vi "IsSearchGoalNode.vi"(8 "error in (no error)":errorcluster, 10 "NodeToIdentify in":refnum<data-value>, 11 "BasicSortedList in":refnum<class "BasicSortedList.lvclass">) -> (0 "error out":errorcluster, 1 "IsNode":bool, 2 "NodeToIdentify out":refnum<data-value>, 3 "BasicSortedList out":refnum<class "BasicSortedList.lvclass">)   [LabVIEW 2009, in "BasicSortedList.lvclass"]
doc: "Determines the goal node of a basic sorted list. If ascending then we check if what we search for is less than the current node. If decending then we check if what we are searching for is greater than the current node."
uses:
  BasicSortedList.lvclass
  LLNode/LLNode.lvclass
  BasicSortedNode/BasicSortedNode.lvclass
  BasicSortedList.lvclass/BasicSortedList.ctl
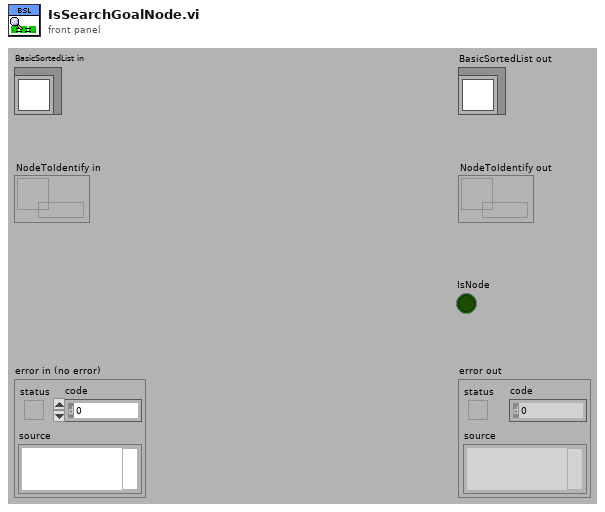
[diagram p1: front panel]
types:
  T1 = typedef "BasicSortedList.lvclass/BasicSortOptions.ctl" = enum16{"Ascending", "Decending"}
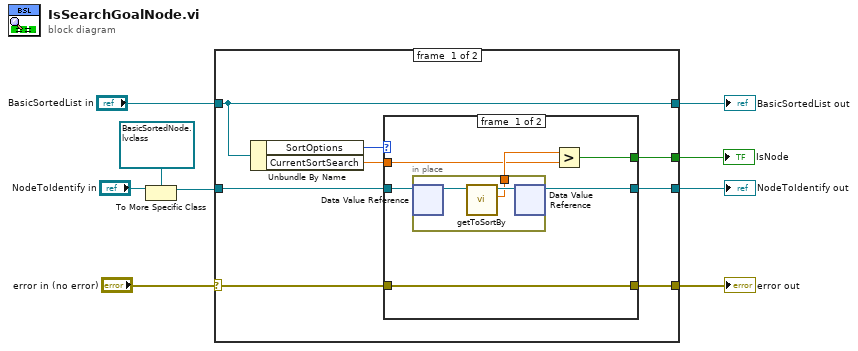
[diagram p0: block diagram]
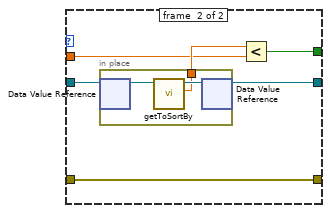
[diagram p2: hidden frame]
diagram:
  n1 = To More Specific Class(target class=refnum<data-value> refnum ("data value reference"), reference="NodeToIdentify in") -> (specific class reference=w5:refnum<data-value>)  [unwired: 1 in, 1 out]
  n2 = case shown="No Error" "error in (no error)" {
    selector: "error in (no error)" -> [w16 w36]
    tunnel: "BasicSortedList in" -> [w13 w38]
    tunnel: w5 -> [w15 w37]
    tunnel: [w13 w38] -> w7
    tunnel: [w12 _] -> w3
    tunnel: [w11 w37] -> w2
    tunnel: [w10 w36] -> w1
    frame #0 {
      n3 = Unbundle By Name(w13) -> ("SortOptions"=w17:T1, "CurrentSortSearch"=w14:dbl)
      n4 = case shown="\"Ascending\", Default" w17 {
        tunnel: w16 -> [w18 w27]
        tunnel: w15 -> [w23 w31]
        tunnel: w14 -> [w21 w29]
        tunnel: [w20 w28] -> w12
        tunnel: [w19 w30] -> w11
        tunnel: [w18 w27] -> w10
        frame #0 {
          n5 = in-place {
            in-place-border: [w24] -> w22
            n6 = in-place-dvr #1(w23) -> (w26:refnum<class "BasicSortedNode.lvclass">)  [unwired: 1 out]
            n7 = call "getToSortBy.vi"("BasicSortedNode in"=w26) -> ("ToSortBy"=w24:dbl, "BasicSortedNode out"=w25:refnum<class "BasicSortedNode.lvclass">)  [unwired: 8 in, 1 out]
            n8 = in-place-dvr #1(w25) -> (w19:refnum<data-value>)  [unwired: 1 out]
          }
          n9 = Greater?(x=w22, y=w21) -> (0:w20:bool)
        }
        frame #1 {
          n10 = in-place {
            in-place-border: [w33] -> w32
            n11 = in-place-dvr #2(w31) -> (w35:refnum<class "BasicSortedNode.lvclass">)  [unwired: 1 out]
            n12 = call "getToSortBy.vi"("BasicSortedNode in"=w35) -> ("ToSortBy"=w33:dbl, "BasicSortedNode out"=w34:refnum<class "BasicSortedNode.lvclass">)  [unwired: 8 in, 1 out]
            n13 = in-place-dvr #2(w34) -> (w30:refnum<data-value>)  [unwired: 1 out]
          }
          n14 = Less?(x=w32, y=w29) -> (x < y?=w28:bool)
        }
      }
    }
    frame #1 {
    }
  }
  "error out" <- w1
  "BasicSortedList out" <- w7
  "NodeToIdentify out" <- w2
  "IsNode" <- w3
